vi "Write FGV Data.vi"(0 "Vision AI in":refnum<class "Vision AI.lvclass">, 1 "0Cv/1St":i32, 5 "DataIn":string, 7 "Data":T1=enum."CurrentAction", 11 "error in (no error)":errorcluster) -> (4 "Vision AI out":refnum<class "Vision AI.lvclass">, 15 "error out":errorcluster)   [LabVIEW 2019, in "Vision AI.lvclass"]
uses:
  Vision AI.lvclass
  Ctrl/Auto Inspection Data Name.ctl
  Ctrl/Auto Inspection Station Name2.ctl
  FlowIOCtrl.lvclass
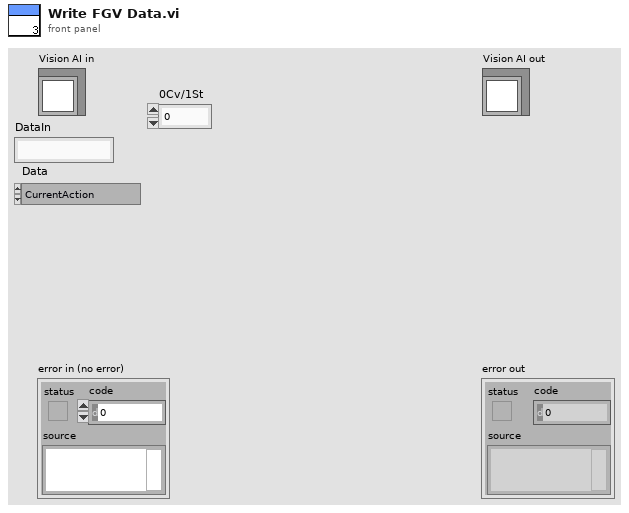
[diagram p1: front panel]
types:
  T1 = typedef "Auto Inspection Data Name.ctl" = enum16{"LocalRun", "ItemSN(TimeCode)", "CurrentAction", "Error", "Data", "OKNG", "電壓值", "電壓值判斷", "電流值", "電流值判斷", "Laser1 Data", "Laser2 Data", "Laser OKNG", "StationNO"}
  T2 = typedef "Auto Inspection Station Name2.ctl" = enum16{"S1Barcode", "S2Measure", "S3Measure", "S4Measure", "S5Measure", "S11_LaserCheck", "S8_Vision AI"}
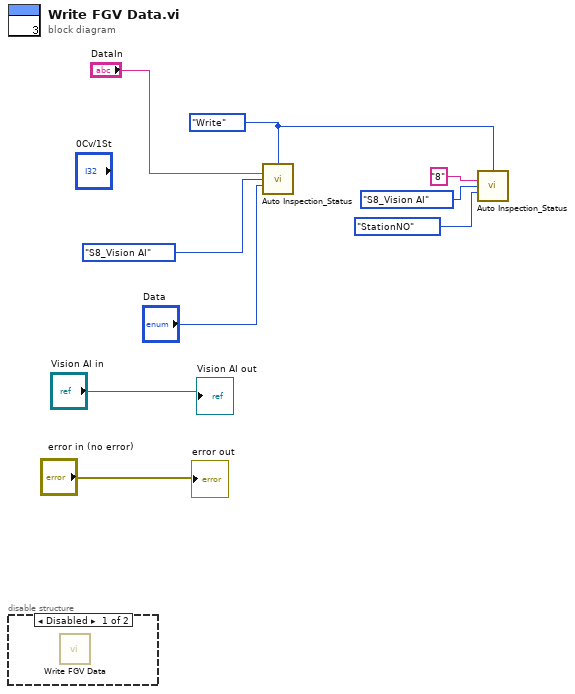
[diagram p0: block diagram]
diagram:
  w7 = enum16{"Initial", "Write", "Read"}."Write" ("Action")
  n1 = disable-structure shown="Disabled" {
    frame Disabled {
      n2 = call-parent "Write FGV Data.vi"() -> ()  [unwired: 14 in, 2 out]
    }
    frame Enabled {
    }
  }
  n3 = call "Auto Inspection_Status.vi"("Action"=w7, "DataIn"="DataIn", "Station"=Auto_Inspection_Station_Name2."S8_Vision AI", "Data"="Data") -> ()  [unwired: 9 in, 3 out]
  n4 = call "Auto Inspection_Status.vi"("Action"=w7, "DataIn"="8", "Station"=Auto_Inspection_Station_Name2."S8_Vision AI", "Data"=Auto_Inspection_Data_Name."StationNO") -> ()  [unwired: 9 in, 3 out]
  "error out" <- "error in (no error)"
  "Vision AI out" <- "Vision AI in"
